vi "Grab images from pco.edge or pco.pixelfly CL.vi"() -> ()   [LabVIEW 2015]
doc: "A short program to demonstrate the fundamentals of control and image acquision with the pco.camera series. The program records a sequence of images, with \"live\" updating, until the \"StopRecording\" button is pressed. Use ctrl-H for more help on the individual controls and indicators.\n\nCopyright 2004, 2010 The Cooke Corporation."
panel:
  out "StorageMode":bool
  out "RecorderSubMode":bool
  out "AcquireEnableInUse":bool
  out "Transfer Parameters":T1
  out "ImageTiming":T2
  out "FrameRate":dbl format="%#.3f"
  out "Waveform Chart":dbl(graph)
  out "cam_fps":dbl=20.079713544692744 caption="FPS" format="%.1g"
  out "bClose":bool
  in  "Quit":bool
  out "BufNr1":i16
  out "BufNr0":i16
  in  "bUseBuffer1":bool
  in  "bUseBuffer0":bool
  in  "ROIX1":u16=1 min=1
  in  "ROIY1":u16=1 min=1
  in  "ROIY0":u16=1 min=1
  in  "ROIX0":u16=1 min=1
  out "Bits/pixel":u16
  in  "Record":bool
  in  "DelayTimeBase":u16(ring)=2 items=["nanoseconds", "microseconds", "milliseconds"]
  in  "ExposureTimeBase":u16(ring)=2 items=["nanoseconds", "microseconds", "milliseconds"]
  in  "Exposure":u32=10
  in  "Delay":u32
  in  "Rate":i32(ring) items=["95333333", "286000000"]
  out "Image":u16[][](graph)
  in  "TriggerMode":u16(ring) items=["Auto", "Software", "External sequence start ", "External exposure control"]
  # "A short program to demonstrate the fundamentals of control and image acquision with the pco.camera series. The program records a sequence of images, with \"live\" updating, until the \"StopRecording\" button is pressed.  Use ctrl-H for more help on the individual controls and indicators."
  # "pco.labview"
  # "1) Setup camera:"
  # "2) Record  images:"
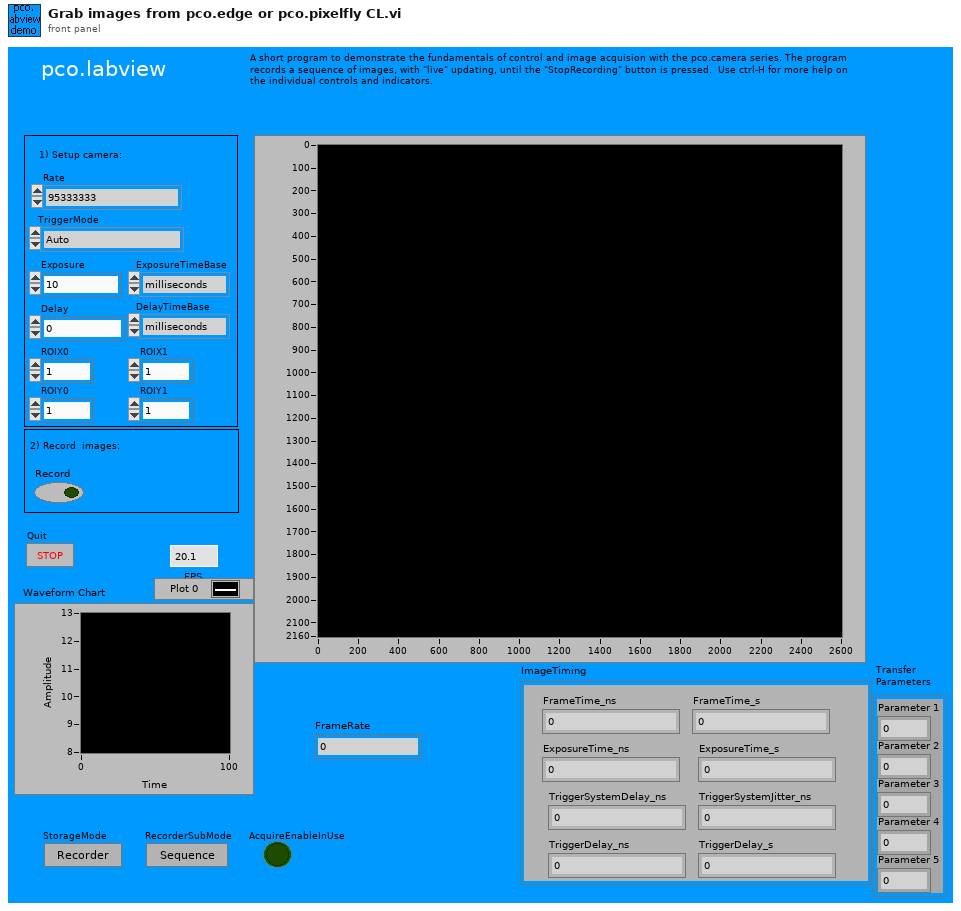
[diagram p1: front panel]
types:
  T1 = cluster{"Parameter 1":u32, "Parameter 2":u32, "Parameter 3":u32, "Parameter 4":u32, "Parameter 5":u32}
  T2 = cluster{"FrameTime_ns":u32, "FrameTime_s":u32, "ExposureTime_ns":u32, "ExposureTime_s":u32, "TriggerSystemDelay_ns":u32, "TriggerSystemJitter_ns":u32, "TriggerDelay_ns":u32, "TriggerDelay_s":u32}
  T3 = cluster{"SSize":u16, "CamType":u16, "CamsSubType":u16, "SerialNumber":u32, "HWVersion":u32, "FWVersion ":u32, "InterfaceType":u16, "HardwareVersions":cluster{"Board":u16, cluster{"string":string, "BatchNumber":u16, "MinorRevision":u8, "MajorRevision":u8, "Variant":u16}[]}, "FirmwareVersions":cluster{"DeviceNum":u16, cluster{"string":string, "MinorRevision":u8, "MajorRevision":u8, "Variant":u16}[]}}
  T4 = cluster{"Size":u16, "SensorTypeDESC":u16, "SensorSubtypeDESC":u16, "MaxHorizontalResStdDESC":u16, "MaxVerticalResStdDESC":u16, "MaxHorizontalResExtDESC":u16, "MaxVerticalResExtDESC":u16, "DynResDESC":u16, "MaxBinHorzDESC":u16, "BinHorzStepDESC":bool, "MaxBinVertDESC":u16, "BinVertStepDESC":bool, "ROIHorzStepDESC":u16, "ROIVertStepDESC":u16, "NumADCDESC":u16, "IRDESC":bool, "MinDelayDESC":u32, "MaxDelayDESC":u32, "MinDelayStepDESC":u32, "MinExpoDESC":u32, "MaxExpoDESC":u32, "MinExpoStepDESC":u32, "MinDelayIRDESC":u32, "MaxDelayIRDESC":u32, "MinExpoIRDESC":u32, "MaxExpoIRDESC":u32, "TimeTableDESC":bool, "DoubleImageDESC":bool, "MinCoolSetDESC":i16, "MaxCoolSetDESC":i16, "MDefaultCoolSetDESC":i16, "PowerDownModeDESC":bool, "OffsetRegDESC":bool, "ColorPattern":cluster{"UpperLeftColor":u8, "UpperRightColor":u8, "LowerLeftColor":u8, "LowerRightColor":u8}, "PatternTypeDESC":bool, "PixelRates":u32[], "CoversionFactors":u16[], "Reserved":u32[], "GeneralCapabilities":u32, "GeneralCapabilities 2":u32, "Min Size Hor":u16, "Min Size Vert":u16, "Ext Synch Freq":u32[], "Cooling Setpoints":i16[], "Soft ROI Hor Step":u16, "Soft ROI Vert Step":u16}
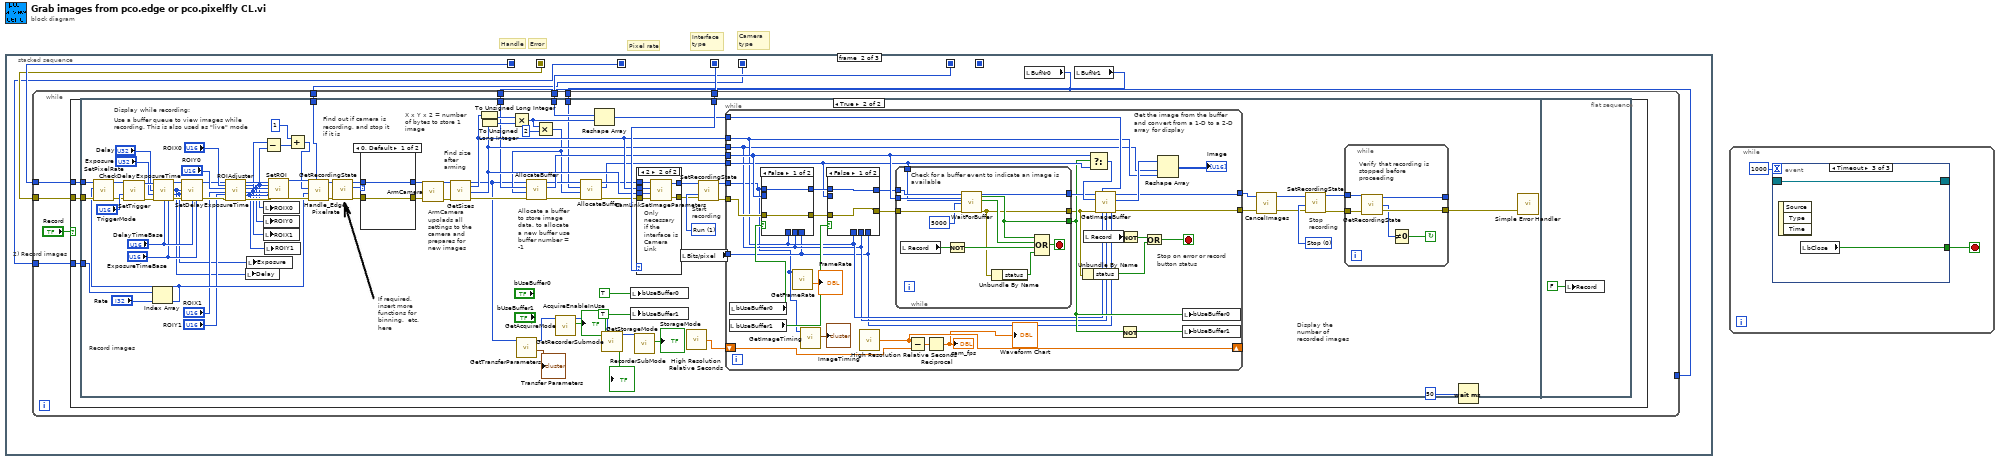
[diagram p0: block diagram]
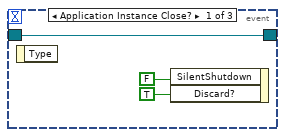
[diagram p2: hidden frame]
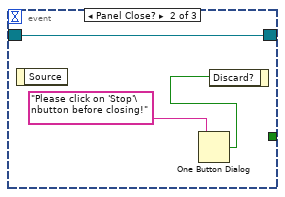
[diagram p3: hidden frame]
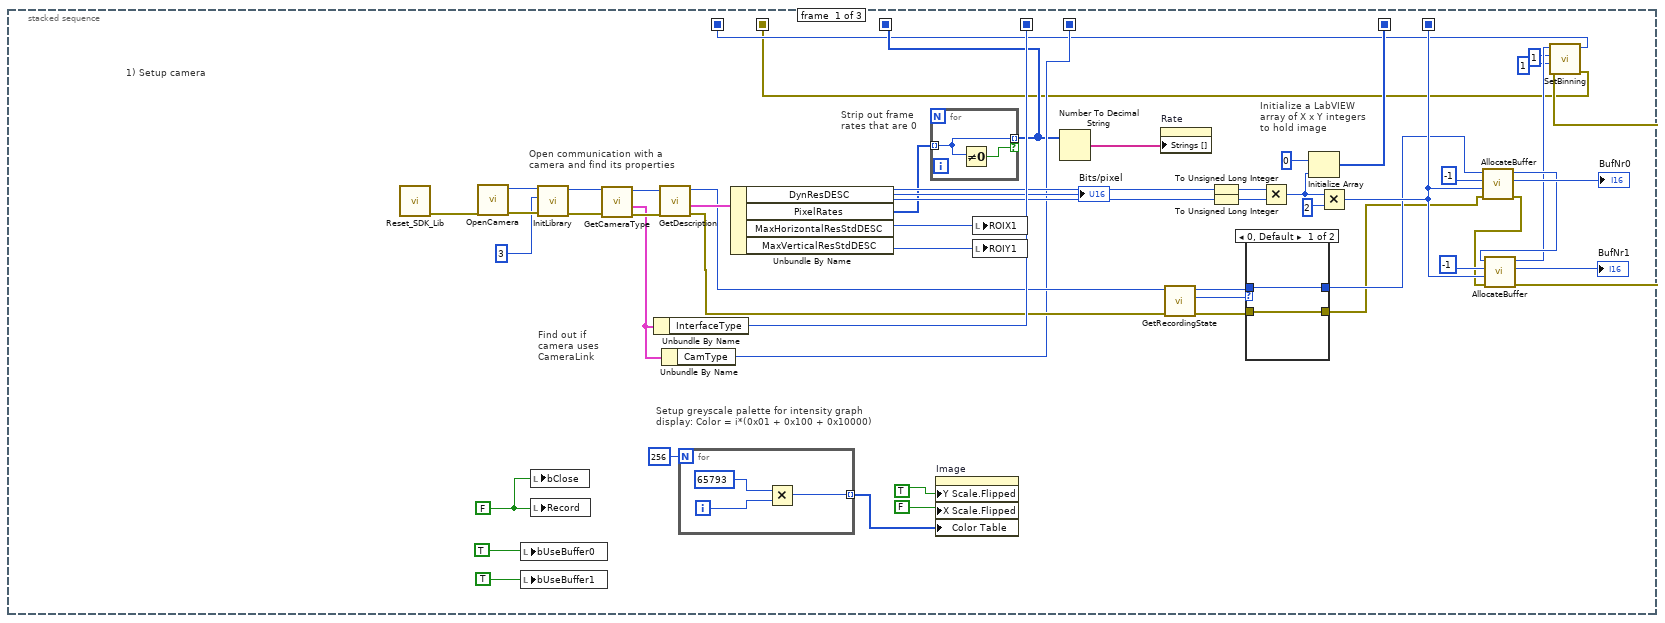
[diagram p4: hidden frame]
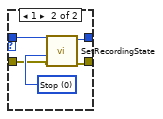
[diagram p5: hidden frame]
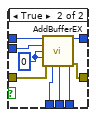
[diagram p7: hidden frame]
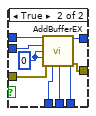
[diagram p8: hidden frame]
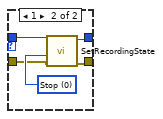
[diagram p10: hidden frame]
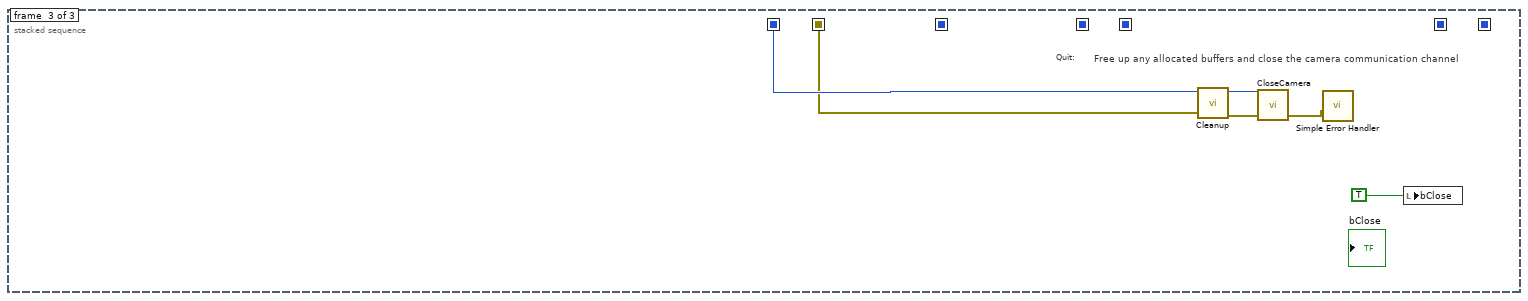
[diagram p11: hidden frame]
diagram:
  # "Camera type"
  # "Interface type"
  # "Error"
  # "Handle"
  # "Pixel rate"
  n1 = stacked-sequence {
    seq-local: [w45 _ _] -> [_ w68 _]
    seq-local: [w33 _ _] -> [_ _ _]
    seq-local: [w5 _ _] -> [_ w71 w271]
    seq-local: [w1 _ _] -> [_ w70 w270]
    seq-local: [w40 _ _] -> [_ w69 _]
    seq-local: [w7 _ _] -> [_ w65 _]
    seq-local: [w9 _ _] -> [_ w64 _]
    frame #0 {
      w27 = FALSE ("stop")
      # "Strip out frame rates that are 0"
      # "1) Setup camera"
      # "Find out if camera uses CameraLink"
      # "Setup greyscale palette for intensity graph display: Color = i*(0x01 + 0x100 + 0x10000)"
      # "Initialize a LabVIEW array of X x Y integers to hold image"
      # "Open communication with a camera and find its properties"
      n2 = call "Reset_SDK_Lib.vi"() -> ("ErrorOut"=w11:errorcluster)  [unwired: 11 in]
      n3 = call "OpenCamera.vi"("ErrorIn"=w11) -> ("ErrorOut"=w24:errorcluster, "Handle out"=w25:u64)  [unwired: 3 in, 2 out]
      n4 = local write "bUseBuffer0"(TRUE) -> ()
      n5 = local write "bUseBuffer1"(TRUE) -> ()
      n6 = local write "bClose"(w27) -> ()
      n7 = local write "Record"(w27) -> ()
      n8 = call "InitLibrary.vi"("error in (no error)"=w24, "InterfaceType"=u32 3, "ph"=w25) -> ("error out"=w23:errorcluster, "hout"=w22:u64)  [unwired: 7 in]
      n9 = call "GetCameraType.vi"("ph"=w22, "error in (no error)"=w23) -> ("hout"=w42:u64, "CameraType"=w10:T3, "error out"=w41:errorcluster)  [unwired: 1 in, 1 out]
      n10 = Unbundle By Name(w10) -> ("InterfaceType"=w40:u16)
      n11 = call "GetDescription.vi"("ErrorIn"=w41, "ph"=w42) -> ("ErrorOut"=w19:errorcluster, "Description"=w44:T4, "hout"=w18:u64)  [unwired: 2 in, 1 out]
      n12 = Unbundle By Name(w10) -> ("CamType"=w9:u16)
      n13 = for {
        N: 256 -> [_]
        tunnel: [w61] -> w48 mode=indexing
        i -> [w62]
        n14 = Multiply(x=65793, y=w62) -> (x*y=w61:i32)
      }
      n15 = Unbundle By Name(w44) -> ("DynResDESC"=→"Bits/pixel":u16, "PixelRates"=w8:u32[], "MaxHorizontalResStdDESC"=w38:u16, "MaxVerticalResStdDESC"=w37:u16)
      n16 = for {
        tunnel: w8 -> [w52] mode=indexing
        tunnel: [w52] -> w7 mode=indexing if=w53
        n17 = Not Equal To 0?(x=w52) -> (x != 0?=w53:bool)
      }
      n18 = property on="Image" class="IntGraph (strict)"("Y Scale.Flipped"=TRUE, "X Scale.Flipped"=FALSE, "Color Table"=w48) -> ()  [unwired: 2 in, 2 out]
      n19 = local write "ROIX1"(w38) -> ()
      n20 = local write "ROIY1"(w37) -> ()
      n21 = Number To Decimal String(number=w7) -> (decimal integer string=w26:string[])  [unwired: 1 in]
      n22 = property on="Rate" class="Ring (strict)"("Strings []"=w26) -> ()  [unwired: 2 in, 2 out]
      n23 = call "GetRecordingState.vi"("ErrorIn"=w19, "ph"=w18) -> ("ErrorOut"=w16:errorcluster, "Error"=w12:i32, "hout"=w17:u64)  [unwired: 2 in, 1 out]
      n24 = To Unsigned Long Integer(number=w38) -> (unsigned 32bit integer=w35:u32)
      n25 = To Unsigned Long Integer(number=w37) -> (unsigned 32bit integer=w34:u32)
      n26 = case shown="0, Default" w12 {
        tunnel: w17 -> [w55 w59]
        tunnel: w16 -> [w54 w58]
        tunnel: [w55 w57] -> w15
        tunnel: [w54 w56] -> w13
        frame 0, Default {
        }
        frame 1 {
          w60 = u16 0 items=["Stop", "Run"] ("RecordingState")
          n27 = call "SetRecordingState.vi"("ErrorIn"=w58, "RecordingState"=w60, "ph"=w59) -> ("ErrorOut"=w56:errorcluster, "hout"=w57:u64)  [unwired: 2 in, 1 out]
        }
      }
      n28 = Multiply(x=w35, y=w34) -> (x*y=w46:u32)
      n29 = Initialize Array(u16 0 ("Element Data"), w46) -> (w45:u16[])
      n30 = Multiply(x=w46, y=u32 2) -> (x*y=w33:u32)
      n31 = call "AllocateBuffer.vi"("error in (no error)"=w13, "Size"=w33, "BufNr"=i16 -1, "ph"=w15) -> ("error out"=w20:errorcluster, "BufNrOut"=→"BufNr0":i16, "hout"=w14:u64)  [unwired: 2 in, 3 out]
      n32 = call "AllocateBuffer.vi"("error in (no error)"=w20, "Size"=w33, "BufNr"=i16 -1, "ph"=w14) -> ("error out"=w2:errorcluster, "BufNrOut"=→"BufNr1":i16, "hout"=w6:u64)  [unwired: 2 in, 3 out]
      n33 = call "SetBinning.vi"("error in (no error)"=w2, "BinVert"=u16 1, "BinHorz"=u16 1, "ph"=w6) -> ("error out"=w1:errorcluster, "hout"=w5:u64)  [unwired: 3 in, 1 out]
    }
    frame #1 {
      n34 = local read "BufNr0"() -> (w67:i16)
      n35 = local read "BufNr1"() -> (w66:i16)
      n36 = while {
        tunnel: w67 -> [_]
        tunnel: w67 -> [w77]
        tunnel: w68 -> [w79]
        tunnel: w69 -> [w80]
        tunnel: w70 -> [w78]
        tunnel: w71 -> [w75]
        tunnel: w66 -> [w76]
        tunnel: w65 -> [w73]
        tunnel: w64 -> [w72]
        stop <- "Quit" stop-if-true
        n37 = case "2) Record images" shown="True" "Record" {
          tunnel: w75 -> [_ w90]
          tunnel: w78 -> [_ w89]
          tunnel: w80 -> [_ w88]
          tunnel: w79 -> [_ w87]
          tunnel: w77 -> [_ w86]
          tunnel: w76 -> [_ w85]
          tunnel: w73 -> [_ w84]
          tunnel: w72 -> [_ w83]
          frame False {
          }
          frame True {
            n38 = flat-sequence {
              tunnel: w90 -> [w164]
              tunnel: w89 -> [w163]
              tunnel: w88 -> [w161]
              tunnel: w87 -> [w159]
              tunnel: w86 -> [w150]
              tunnel: w85 -> [w144]
              tunnel: w84 -> [w131]
              tunnel: w83 -> [w122]
              frame #0 {
                w176 = u16 1 items=["Stop", "Run"] ("RecordingState")
                w179 = u16 0 items=["Stop", "Run"] ("RecordingState")
                # "Display the number of recorded images"
                # "Record images"
                # "Start recording"
                # "Allocate a buffer to store image data. to allocate a new buffer use buffer number = -1"
                # "Find size after arming"
                # "ArmCamera upolads all settings to the camera and prepares for new images"
                # "Find out if camera is recording, and stop it if it is"
                # "If required, insert more functions for binning.  etc. here"
                # "X x Y x 2 = number of bytes to store 1 image"
                # "Stop recording"
                # "Use a buffer queue to view images while recording. This is also used as \"live\" mode"
                # "Display while recording:"
                n39 = Index Array(array=w131, index="Rate") -> (element=w126:u32)
                n40 = call "SetPixelRate.vi"("error in (no error)"=w163, "PixelRate"=w126, "ph"=w164) -> ("error out"=w133:errorcluster, "hout"=w134:u64)  [unwired: 2 in, 1 out]
                n41 = call "SetTrigger.vi"("error in (no error)"=w133, "TriggerMode"="TriggerMode", "ph"=w134) -> ("error out"=w107:errorcluster, "hout"=w109:u64)  [unwired: 2 in, 1 out]
                n42 = call "CheckDelayExposureTime.vi"("ph"=w109, "Delay"="Delay", "Exposure"="Exposure", "error in (no error)"=w107, "DelayTimeBase"="DelayTimeBase", "ExposureTimeBase"="ExposureTimeBase") -> ("hout"=w108:u64, "Delay Out"=w101:u32, "Exposure Out"=w100:u32, "error out"=w102:errorcluster)  [unwired: 4 in, 2 out]
                n43 = call "SetDelayExposureTime.vi"("ph"=w108, "Delay"=w101, "Exposure"=w100, "error in (no error)"=w102, "DelayTimeBase"="DelayTimeBase", "ExposureTimeBase"="ExposureTimeBase") -> ("hout"=w115:u64, "error out"=w121:errorcluster)  [unwired: 7 in, 1 out]
                n44 = call "ROIAdjuster.vi"("HandleIn"=w115, "ROIXmin"="ROIX0", "ROIYmin"="ROIY0", "ROIXmax"="ROIX1", "ROIYmax"="ROIY1", "ErrorIn"=w121) -> ("hout"=w114:u64, "ROIX0Mod"=w110:u16, "ROIY0Mod"=w111:u16, "ROIX1Mod"=w112:u16, "ROIY1Mod"=w113:u16, "ErrorOut"=w120:errorcluster)  [unwired: 7 in, 1 out]
                n45 = local write "Delay"(w101) -> ()
                n46 = local write "Exposure"(w100) -> ()
                n47 = Subtract(x=w112, y=w110) -> (x-y=w125:u16)
                n48 = local write "ROIX0"(w110) -> ()
                n49 = local write "ROIY0"(w111) -> ()
                n50 = local write "ROIX1"(w112) -> ()
                n51 = local write "ROIY1"(w113) -> ()
                n52 = call "SetROI.vi"("ph"=w114, "ROIX0"=w110, "ROIY0"=w111, "ROIX1"=w112, "ROIY1"=w113, "error in (no error)"=w120) -> ("hout"=w127:u64, "error out"=w128:errorcluster)  [unwired: 12 in]
                n53 = Add(x=1, y=w125) -> (x+y=w123:i32)
                n54 = call "Handle_Edge_Pixelrate.vi"("Cameratype"=w122, "error in (no error)"=w128, "PixelRate"=w126, "X-Resolution"=w123, "ph"=w127) -> ("error out"=w129:errorcluster, "hout"=w130:u64)  [unwired: 5 in]
                n55 = call "GetRecordingState.vi"("ErrorIn"=w129, "ph"=w130) -> ("ErrorOut"=w173:errorcluster, "RecordingState"=w175:u16, "hout"=w174:u64)  [unwired: 2 in, 1 out]
                n56 = case shown="0, Default" w175 {
                  tunnel: w174 -> [w263 w267]
                  tunnel: w173 -> [w262 w266]
                  tunnel: [w263 w265] -> w172
                  tunnel: [w262 w264] -> w171
                  frame 0, Default {
                  }
                  frame 1 {
                    w268 = u16 0 items=["Stop", "Run"] ("RecordingState")
                    n57 = call "SetRecordingState.vi"("ErrorIn"=w266, "RecordingState"=w268, "ph"=w267) -> ("ErrorOut"=w264:errorcluster, "hout"=w265:u64)  [unwired: 2 in, 1 out]
                  }
                }
                n58 = call "ArmCamera.vi"("error in (no error)"=w171, "ph"=w172) -> ("error out"=w169:errorcluster, "hout"=w170:u64)  [unwired: 1 in, 1 out]
                n59 = call "GetSizes.vi"("ph"=w170, "ErrorIn"=w169) -> ("hout"=w98:u64, "XResAct"=w157:u16, "YResAct"=w156:u16, "ErrorOut"=w168:errorcluster)  [unwired: 11 in, 3 out]
                n60 = To Unsigned Long Integer(number=w157) -> (unsigned 32bit integer=w151:u32)
                n61 = To Unsigned Long Integer(number=w156) -> (unsigned 32bit integer=w152:u32)
                n62 = Multiply(x=w151, y=w152) -> (x*y=w153:u32)
                n63 = call "GetTransferParameters.vi"("ph"=w98) -> ("Transfer Parameters"=→"Transfer Parameters":T1, "hout"=w97:u64)  [unwired: 3 in, 2 out]
                n64 = Multiply(x=w153, y=u32 2) -> (x*y=w145:u32)
                n65 = call "AllocateBuffer.vi"("error in (no error)"=w168, "Size"=w145, "BufNr"=w150, "ph"=w98) -> ("error out"=w149:errorcluster, "BufNrOut"=w154:i16, "hout"=w147:u64)  [unwired: 2 in, 3 out]
                n66 = call "GetAcquireMode.vi"("ph"=w97) -> ("AcquireEnableInUse"=→"AcquireEnableInUse":bool, "hout"=w96:u64)  [unwired: 3 in, 2 out]
                n67 = call "AllocateBuffer.vi"("error in (no error)"=w149, "Size"=w145, "BufNr"=w144, "ph"=w147) -> ("error out"=w148:errorcluster, "BufNrOut"=w143:i16, "hout"=w146:u64)  [unwired: 2 in, 3 out]
                n68 = Reshape Array(w159, w153) -> (w158:u16[])
                n69 = call "GetRecorderSubmode.vi"("ph"=w96) -> ("RecorderSubMode"=→"RecorderSubMode":bool, "hout"=w95:u64)  [unwired: 3 in, 2 out]
                n70 = local write "bUseBuffer0"(TRUE) -> ()
                n71 = local write "bUseBuffer1"(TRUE) -> ()
                n72 = call "GetStorageMode.vi"("ph"=w95) -> ("StorageMode"=→"StorageMode":bool)  [unwired: 3 in, 3 out]
                n73 = case shown="2" w161 {
                  tunnel: w148 -> [w254 w261]
                  tunnel: [w254 w260] -> w166
                  tunnel: w146 -> [w255 w259]
                  tunnel: [w255 w258] -> w165
                  tunnel: w156 -> [_ w257]
                  tunnel: w157 -> [_ w256]
                  frame 0, Default {
                  }
                  frame 2 {
                    # "Only necessary if the interface is Camera Link"
                    n74 = call "CamLinkSetImageParameters.vi"("error in (no error)"=w261, "YRes"=w257, "XRes"=w256, "ph"=w259) -> ("error out"=w260:errorcluster, "hout"=w258:u64)  [unwired: 1 out]
                  }
                }
                n75 = local read "Bits/pixel"() -> (w138:u16)
                n76 = call <vilib>:"High Resolution Relative Seconds.vi"() -> ("relative seconds"=w99:dbl)
                n77 = call "SetRecordingState.vi"("ErrorIn"=w166, "RecordingState"=w176, "ph"=w165) -> ("ErrorOut"=w162:errorcluster, "hout"=w160:u64)  [unwired: 2 in, 1 out]
                n78 = while {
                  tunnel: w154 -> [w199]
                  tunnel: w158 -> [w208]
                  tunnel: w160 -> [w181]
                  tunnel: w156 -> [w188]
                  tunnel: w157 -> [w189]
                  tunnel: w162 -> [w206]
                  tunnel: [w210] -> w137
                  tunnel: [w211] -> w136
                  tunnel: w143 -> [w198]
                  tunnel: w138 -> [w187]
                  shift-right: [w184] -> _
                  shift-left: w99 -> [w185]
                  stop <- w190 stop-if-true
                  # "Stop on error or record button status"
                  # "Get the image from the buffer and convert from a 1-D to a 2-D array for display"
                  n79 = local read "bUseBuffer1"() -> (w203:bool)
                  n80 = local read "bUseBuffer0"() -> (w204:bool)
                  n81 = case shown="False" w204 {
                    tunnel: [w214 w223] -> w205
                    tunnel: [w213 w222] -> w207
                    tunnel: w199 -> [_ w221]
                    tunnel: w181 -> [w213 w220]
                    tunnel: w187 -> [_ w218]
                    tunnel: w189 -> [_ w217]
                    tunnel: w188 -> [_ w216]
                    tunnel: w206 -> [w214 w215]
                    frame False {
                    }
                    frame True {
                      w219 = i16 0
                      n82 = call "AddBufferEX.vi"("ph"=w220, "BuffNr"=w221, "1stImage"=w219, "LastImage"=w219, "error in (no error)"=w215, "XRes"=w217, "YRes"=w216, "BitPerPixel"=w218) -> ("hout"=w222:u64, "error out"=w223:errorcluster)  [unwired: 5 in, 1 out]
                    }
                  }
                  n83 = call "GetFrameRate.vi"("ph"=w181) -> ("FrameRate"=→"FrameRate":dbl)  [unwired: 3 in, 5 out]
                  n84 = call "GetImageTiming.vi"("ph"=w181) -> ("ImageTiming"=→"ImageTiming":T2)  [unwired: 4 in, 3 out]
                  n85 = case shown="False" w203 {
                    tunnel: [w224 w234] -> w196
                    tunnel: [w225 w233] -> w197
                    tunnel: w198 -> [_ w232]
                    tunnel: w207 -> [w225 w231]
                    tunnel: w187 -> [_ w229]
                    tunnel: w189 -> [_ w228]
                    tunnel: w188 -> [_ w227]
                    tunnel: w205 -> [w224 w226]
                    frame False {
                    }
                    frame True {
                      w230 = i16 0
                      n86 = call "AddBufferEX.vi"("ph"=w231, "BuffNr"=w232, "1stImage"=w230, "LastImage"=w230, "error in (no error)"=w226, "XRes"=w228, "YRes"=w227, "BitPerPixel"=w229) -> ("hout"=w233:u64, "error out"=w234:errorcluster)  [unwired: 5 in, 1 out]
                    }
                  }
                  n87 = call <vilib>:"High Resolution Relative Seconds.vi"() -> ("relative seconds"=w184:dbl)
                  n88 = while {
                    tunnel: w199 -> [w242]
                    tunnel: w198 -> [w241]
                    tunnel: w197 -> [w244]
                    tunnel: w196 -> [w243]
                    tunnel: [w240] -> w195
                    tunnel: [w236] -> w193
                    tunnel: [w239] -> w194
                    stop <- w245 stop-if-true
                    # "Check for a buffer event to indicate an image is available"
                    n89 = local read "Record"() -> (w247:bool)
                    n90 = Not(x=w247) -> (.not. x?=w246:bool)
                    n91 = call "WaitForBuffer.vi"("ph"=w244, "sBufNr"=w242, "sBufNr 2"=w241, "timeout"=5000, "error in (no error)"=w243) -> ("hout"=w240:u64, "Buffer_Ready"=w239:bool, "Buffer_Ready 2"=w238:bool, "error out"=w236:errorcluster)  [unwired: 10 in, 1 out]
                    n92 = Unbundle By Name(w236) -> ("status"=w235:bool)
                    n93 = Compound Arithmetic op=OR(w239, w238, w246, w235) -> (w245:bool)
                  }
                  n94 = Subtract(x=w184, y=w185) -> (x-y=w186:dbl)
                  n95 = Reciprocal(x=w186) -> (1/x=→"cam_fps" →"Waveform Chart":dbl)
                  n96 = Unbundle By Name(w193) -> ("status"=w191:bool)
                  n97 = local read "Record"() -> (w209:bool)
                  n98 = Select(t=w199, s=w194, f=w198) -> (s? t:f=w202:i16)
                  n99 = call "GetImageBuffer.vi"("ph"=w195, "BuffIn"=w208, "BuffNr"=w202, "error in (no error)"=w193, "xRes"=w189, "yRes"=w188, "Bitresolution"=w187) -> ("hout"=w210:u64, "BuffOut"=w212:u16[], "error out"=w211:errorcluster)  [unwired: 5 in, 1 out]
                  n100 = Not(x=w194) -> (.not. x?=w201:bool)
                  n101 = Not(x=w209) -> (.not. x?=w192:bool)
                  n102 = Or(x=w192, y=w191) -> (x .or. y?=w190:bool)
                  n103 = Reshape Array(w212, w188, w189) -> (→"Image":u16[][])
                  n104 = local write "bUseBuffer0"(w194) -> ()
                  n105 = local write "bUseBuffer1"(w201) -> ()
                }
                n106 = call "CancelImages.vi"("error in (no error)"=w136, "ph"=w137) -> ("error out"=w140:errorcluster, "hout"=w139:u64)  [unwired: 1 in, 1 out]
                n107 = call "SetRecordingState.vi"("ErrorIn"=w140, "RecordingState"=w179, "ph"=w139) -> ("ErrorOut"=w177:errorcluster, "hout"=w178:u64)  [unwired: 2 in, 1 out]
                n108 = while {
                  tunnel: [w251] -> w135
                  tunnel: w177 -> [w252]
                  tunnel: w178 -> [w253]
                  tunnel: [w248] -> _
                  stop <- w249 continue-if-true
                  # "Verify that recording is stopped before proceeding"
                  n109 = call "GetRecordingState.vi"("ErrorIn"=w252, "ph"=w253) -> ("ErrorOut"=w251:errorcluster, "RecordingState"=w250:u16, "hout"=w248:u64)  [unwired: 2 in, 1 out]
                  n110 = Not Equal To 0?(x=w250) -> (x != 0?=w249:bool)
                }
                n111 = call <vilib>:"Simple Error Handler.vi"("error in (no error)"=w135) -> ()  [unwired: 4 in, 5 out]
              }
              frame #1 {
                n112 = local write "Record"(FALSE ("Record")) -> ()
              }
            }
          }
        }
        n113 = Wait (ms)(milliseconds to wait=u32 50) -> ()  [unwired: 1 out]
      }
    }
    frame #2 {
      # "Free up any allocated buffers and close the camera communication channel"
      # "Quit:"
      n114 = call "Cleanup.vi"("error in (no error)"=w270, "ph"=w271) -> ("error out"=w272:errorcluster, "hout"=w273:u64)  [unwired: 8 in]
      n115 = call "CloseCamera.vi"("ErrorIn"=w272, "Handle in"=w273) -> ("ErrorOut"=w275:errorcluster)  [unwired: 1 in, 2 out]
      n116 = call <vilib>:"Simple Error Handler.vi"("error in (no error)"=w275) -> ()  [unwired: 4 in, 5 out]
      n117 = local write "bClose"(TRUE) -> ()
    }
  }
  n118 = while {
    stop <- w276 stop-if-true
    n119 = event shown="[2] Timeout" {
      selector: _ -> [w278 w283 w285]
      dyn-events: [w278 w283 w285] -> _
      timeout: 1000 -> [_ _ _]
      tunnel: [_ _ w284] -> w276
      event Application Instance Close? {
        n120 = event-data() -> ()  [unwired: 1 in, 1 out]
        n121 = event-data("SilentShutdown"=FALSE, "Discard?"=TRUE) -> ()  [unwired: 1 in, 1 out]
      }
      event Panel Close? {
        n122 = event-data() -> ()  [unwired: 1 in, 1 out]
        n123 = One Button Dialog(message="Please click on 'Stop'\nbutton before closing!") -> (true=w281:bool)  [unwired: 1 in]
        n124 = event-data("Discard?"=w281) -> ()  [unwired: 1 in, 1 out]
      }
      event Timeout {
        n125 = event-data() -> ()  [unwired: 1 in, 3 out]
        n126 = local read "bClose"() -> (w284:bool)
      }
    }
  }
